vi "AMC Destroy Message Queue.vi"(8 "error in (no error)":errorcluster, 11 "Message Queue in":T1) -> (0 "error out":errorcluster, 3 "Queue Name":string)   [LabVIEW 2015]
doc: "This VI is used for compatibility with previous versions of the AMC library. Use the AMC VIs located in the <b>Data Communication >> Asynchronous Message Communication</b> palette."
uses:
  <vilib>/NI/AMC/Message Queue.ctl
  <vilib>/NI/AMC/Message.ctl
  <vilib>/NI/Tools/Keyed Array/KeyedArray.ctl
  <vilib>/NI/AMC/AMC.lvlib
  <vilib>/NI/Tools/Keyed Array/Tools_KeyedArray.lvlib
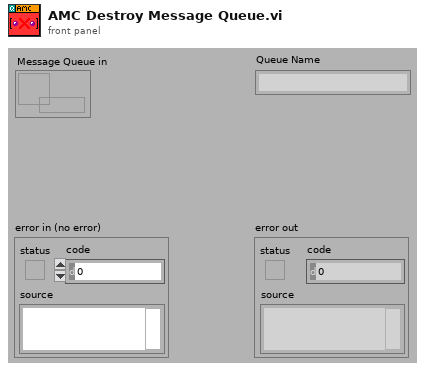
[diagram p1: front panel]
types:
  T1 = typedef "AMC.lvlib/Message Queue.ctl" = refnum<queue>
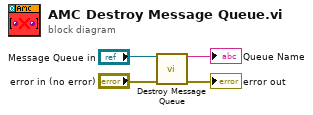
[diagram p0: block diagram]
diagram:
  n1 = call <vilib>:"Destroy Message Queue.vi"("message queue in"="Message Queue in", "error in"="error in (no error)") -> ("message queue name"=→"Queue Name":string, "error out"=→"error out":errorcluster)  [unwired: 11 in, 1 out]
